vi "read TBM configuration.vi"(8 "error in":errorcluster, 11 "fixed module parent implementation editor node in":refnum<class "fixed channel editor.lvclass">) -> (0 "error out":errorcluster, 2 "configuration":refnum<class "TBM configuration.lvclass">, 3 "fixed module parent implementation editor node out":refnum<class "fixed channel editor.lvclass">)   [LabVIEW 2013, in "fixed channel editor.lvclass"]
uses:
  fixed channel editor.lvclass
  <vilib>/NI/Tag Bus Module Framework/root configuration/TBM configuration.lvclass
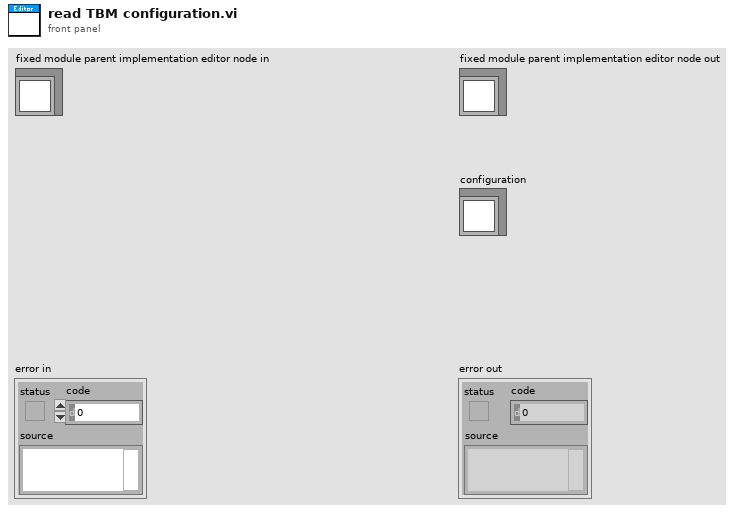
[diagram p1: front panel]
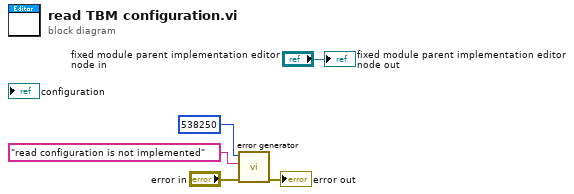
[diagram p0: block diagram]
diagram:
  n1 = call <vilib>:"error generator.vi"("error in"="error in", "append error message"="read configuration is not implemented", "error code (0)"=538250) -> ("error out"=→"error out":errorcluster)  [unwired: 8 in]
  "fixed module parent implementation editor node out" <- "fixed module parent implementation editor node in"
